vi "Lint Class.vi"(8 "Error In":errorcluster, 10 "Results In":T1[](array[typedef]), 11 "Project Item In":refnum<vi>) -> (0 "Error Out":errorcluster, 2 "Results Out":T1[](array[typedef]), 3 "Project Item Out":refnum<vi>)   [LabVIEW 2018, in "Scripts.lvlib"]
uses:
  Scripts.lvlib
  Project Item Lint Result.ctl
  VI Control Lint Result.ctl
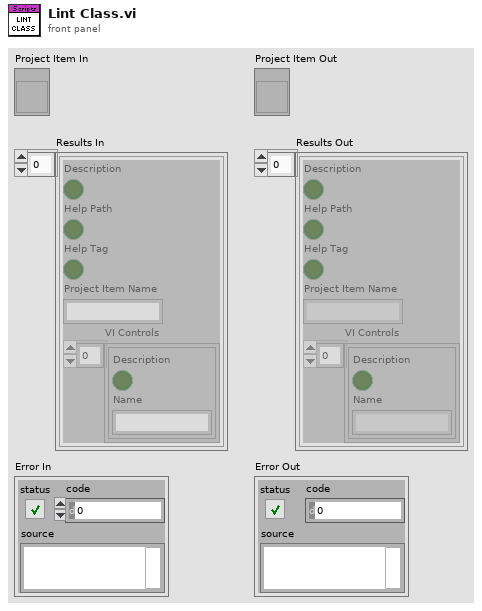
[diagram p1: front panel]
types:
  T1 = typedef "Scripts.lvlib/Project Item Lint Result.ctl" = cluster{"Description":bool, "Help Path":bool, "Help Tag":bool, "Project Item Name":string, "VI Controls":T2[]}
  T2 = typedef "Scripts.lvlib/VI Control Lint Result.ctl" = cluster{"Description":bool, "Name":string}
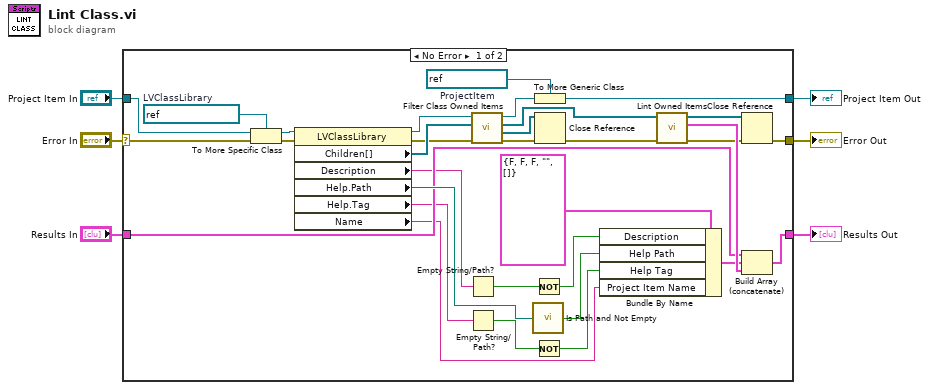
[diagram p0: block diagram]
diagram:
  n1 = case shown="No Error" "Error In" {
    selector: "Error In" -> [w7 w40]
    tunnel: [w36 w39] -> w6
    tunnel: "Results In" -> [w33 w39]
    tunnel: [w22 w41] -> w4
    tunnel: "Project Item In" -> [w16 w41]
    tunnel: [w15 w40] -> w2
    frame No Error {
      w23 = refnum<vi> refnum  # ProjectItem
      w17 = refnum<vi> refnum  # LVClassLibrary
      n2 = To More Specific Class(target class=w17, reference=w16, error in=w7) -> (specific class reference=w18:refnum<vi>, error out=w20:errorcluster)
      n3 = property class="LVClassLibrary"(reference=w18, error in=w20) -> (reference out=w19:refnum<vi>, error out=w21:errorcluster, "Children[]"=w32:refnum<vi>[], "Description"=w31:string, "Help.Path"=w37:path, "Help.Tag"=w24:string, "Name"=w28:string)
      n4 = Empty String/Path?(string/path=w31) -> (empty?=w26:bool)
      n5 = Empty String/Path?(string/path=w24) -> (empty?=w27:bool)
      n6 = call "Filter Class Owned Items.vi"("Error In"=w21, "Children[]"=w32, "LVClassLibrary In"=w19) -> ("Error Out"=w10:errorcluster, "Private Items"=w9:refnum<vi>[], "Non-Private Items"=w11:refnum<vi>[], "LVClassLibrary Out"=w8:refnum<vi>)  [unwired: 5 in]
      n7 = call <vilib>:"Is Path and Not Empty.vi"("path"=w37) -> ("Is Path and Not Empty?"=w38:bool)  [unwired: 4 in]
      n8 = Not(x=w26) -> (.not. x?=w29:bool)
      n9 = Not(x=w27) -> (.not. x?=w30:bool)
      n10 = To More Generic Class(target class=w23, reference=w8) -> (generic class reference=w22:refnum<vi>)
      n11 = Close Reference(reference=w9, error in (no error)=w10) -> (error out=w12:errorcluster)
      n12 = Bundle By Name(cluster=T1 {"Description"=FALSE, "Help Path"=FALSE, "Help Tag"=FALSE, "Project Item Name"="", "VI Controls"=[]} ("Lint Result"), "Description"=w29, "Help Path"=w38, "Help Tag"=w30, "Project Item Name"=w28) -> (w34:T1)
      n13 = call "Lint Owned Items.vi"("Error In"=w12, "Owned Items In"=w11) -> ("Error Out"=w14:errorcluster, "Results"=w35:T1[], "Owned Items Out"=w13:refnum<vi>[])  [unwired: 7 in]
      n14 = Close Reference(reference=w13, error in (no error)=w14) -> (error out=w15:errorcluster)
      n15 = Build Array (concatenate)(w33, w34, w35) -> (w36:T1[])
    }
    frame Error {
    }
  }
  "Results Out" <- w6
  "Project Item Out" <- w4
  "Error Out" <- w2
